vi "XY Graph Save Selected Plots Event.vi"(6 "Delimiter (TAB)":string="\t", 7 "X Axis Option (Dialog)":T1(ring), 8 "Error In":errorcluster, 9 "Save All Plots? (T)":bool=TRUE, 10 "File Path in":path, 11 "XYGraph Ref":T2) -> (0 "Error Out":errorcluster, 1 "Message":string, 2 "File Path out":path, 3 "Saved Plot Names":string[](array[string]), 4 "Saved Plot Indices":i32[](array[numeric]), 5 "Graph Name":string)   [LabVIEW 2021, in "XY Graph Add-Ons.lvlib"]
uses:
  XY Graph Add-Ons.lvlib
  XY Graph Refnum.ctl
  <userlib>/_OpenG.lib/array/array.llb/Index 1D Array Elements (Variant)__ogtk.vi
  <userlib>/_OpenG.lib/string/string.llb/openg_string.lvlib
  Strings/Strings.lvlib
  <userlib>/_OpenG.lib/array/array.llb/openg_array.lvlib
  GUI/GUI.lvlib
  Files/Files.lvlib
  Utilities/Utilities.lvlib
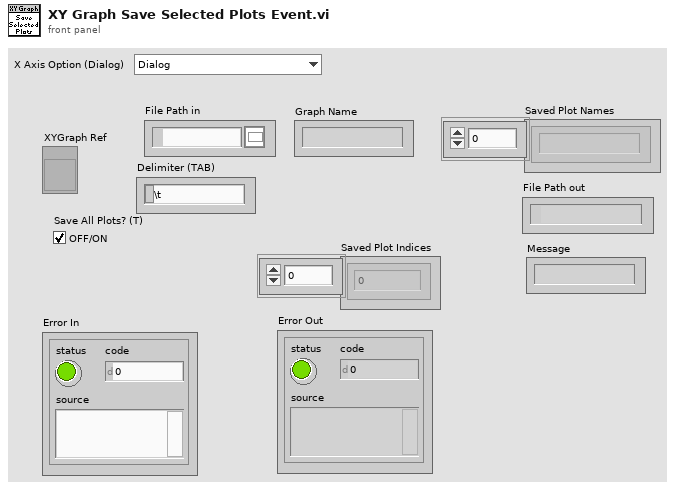
[diagram p1: front panel]
types:
  T1 = enum16{"Dialog", "Save Single X Axis if Common", "Save X Axis for each Plot"}
  T2 = typedef "XY Graph Add-Ons.lvlib/XY Graph Refnum.ctl" = refnum<vi>
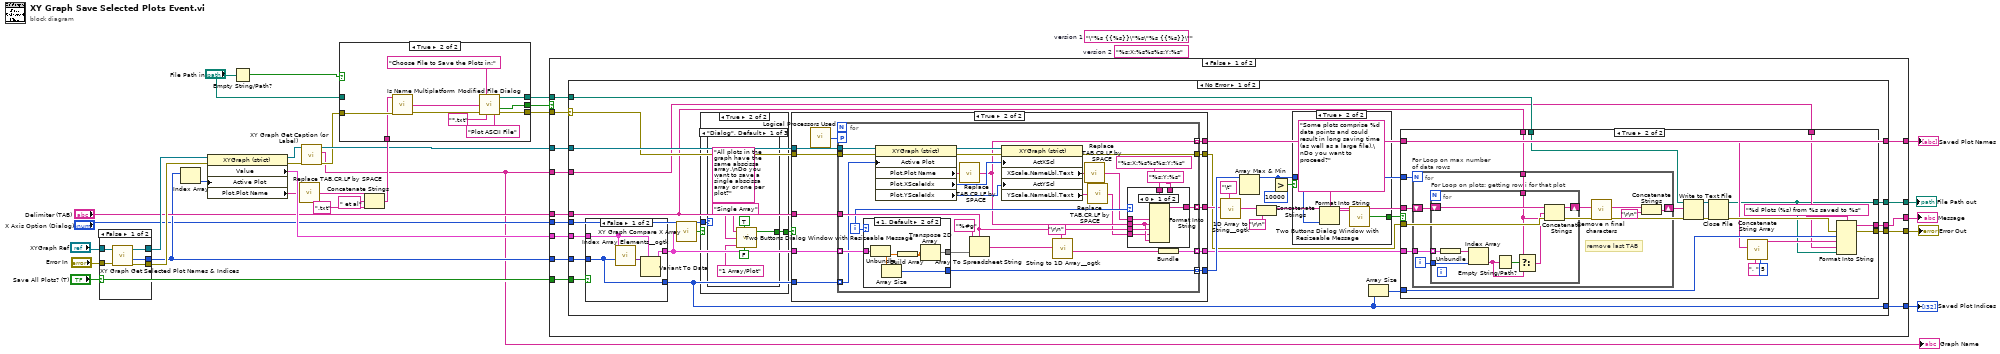
[diagram p0: block diagram]
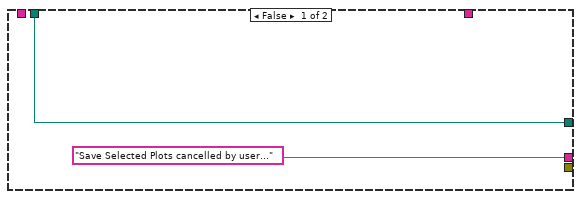
[diagram p2: hidden frame]
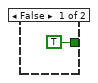
[diagram p3: hidden frame]
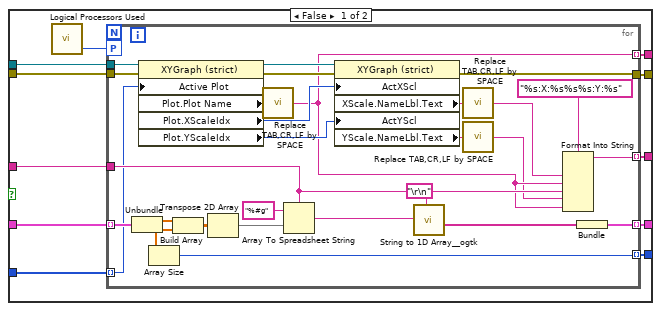
[diagram p4: hidden frame]
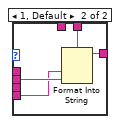
[diagram p5: hidden frame]
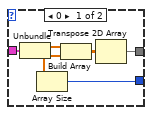
[diagram p6: hidden frame]
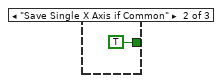
[diagram p8: hidden frame]
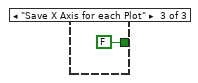
[diagram p9: hidden frame]
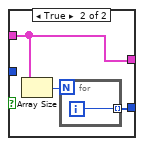
[diagram p10: hidden frame]
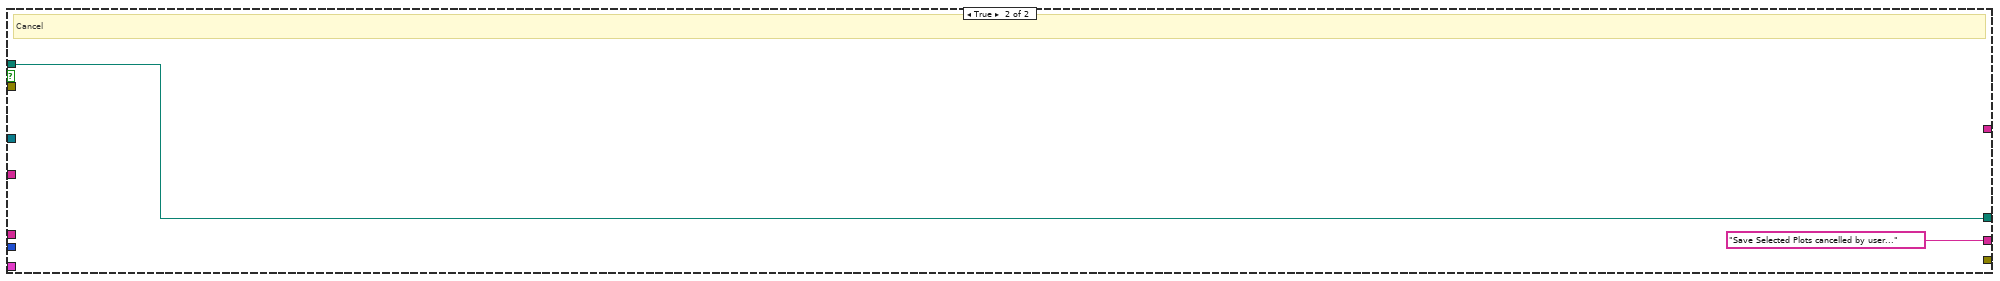
[diagram p12: hidden frame]
diagram:
  (unwired) "%s:X:%s%s%s:Y:%s"  # version 2
  (unwired) "\"%s {{%s}}\"%s\"%s {{%s}}\""  # version 1
  n1 = case shown="False" "Save All Plots? (T)" {
    tunnel: "XYGraph Ref" -> [w35 w37]
    tunnel: "Error In" -> [w34 w36]
    tunnel: [w33 w37] -> w28
    tunnel: [w32 _] -> w16
    tunnel: [w31 w36] -> w23
    frame False {
      n2 = call "XY Graph Get Selected Plot Names & Indices.vi"("error in (no error)"=w34, "XYGraph in"=w35) -> ("error out"=w31:errorcluster, "Selected Plots"=w32:i32[], "XYGraph out"=w33:T2)  [unwired: 5 in, 2 out]
    }
    frame True {
    }
  }
  n3 = Index Array(array=w16) -> (element=w15:i32)  [unwired: 1 in]
  n4 = property class="XYGraph (strict)"(reference=w28, error in=w23, "Active Plot"=w15) -> (reference out=w26:T2, error out=w5:errorcluster, "Value"=w27:cluster{"X Array":dbl[], "Y Array":dbl[]}[], "Plot.Plot Name"=w14:string)
  n5 = Empty String/Path?(string/path="File Path in") -> (empty?=w10:bool)
  n6 = call "Replace TAB,CR,LF by SPACE.vi"("String"=w14) -> ("String with replacements"=w1:string)  [unwired: 8 in]
  n7 = call "XY Graph Get Caption (or Label).vi"("error in (no error)"=w5, "XYGraph in"=w26) -> ("error out"=w4:errorcluster, "Caption (or Label) Text"=w3:string, "XYGraph out"=w6:T2)  [unwired: 7 in]
  "Graph Name" <- w3
  n8 = Concatenate Strings(w1, " et al" ("string"), ".txt" ("string")) -> (w11:string)
  n9 = case shown="True" w10 {
    tunnel: [w38 w49] -> w22
    tunnel: [w39 w48] -> w21
    tunnel: w4 -> [w38 w47]
    tunnel: w11 -> [_ w45]
    tunnel: "File Path in" -> [w39 _]
    tunnel: [_ w43] -> w2
    frame False {
    }
    frame True {
      n10 = call <vilib>:"Is Name Multiplatform.vi"("error in (no error)"=w47, "filename"=w45) -> ("error out"=w46:errorcluster, "suggested filename"=w44:string)  [unwired: 5 in, 3 out]
      n11 = call "Modified File Dialog.vi"("prompt"="Choose File to Save the Plots in:", "suggested filename"=w44, "error in (no error)"=w46, "pattern"="*.txt" ("pattern (all files)"), "pattern label"="Plot ASCII File") -> ("selected path"=w48:path, "Cancelled"=w43:bool, "error out"=w49:errorcluster)  [unwired: 7 in, 1 out]
    }
  }
  n12 = case shown="False" w2 {
    tunnel: w27 -> [w63 _]
    tunnel: [w62 _] -> w25
    tunnel: [w61 _] -> w24
    tunnel: w22 -> [w60 _]
    tunnel: w21 -> [w59 w257]
    tunnel: [w58 w257] -> w20
    tunnel: "Save All Plots? (T)" -> [w57 _]
    tunnel: [w56 _] -> w18
    tunnel: "Delimiter (TAB)" -> [w55 _]
    tunnel: w16 -> [w54 _]
    tunnel: "X Axis Option (Dialog)" -> [w53 _]
    tunnel: [w52 "Save Selected Plots cancelled by user..."] -> w7
    tunnel: w6 -> [w51 _]
    tunnel: w3 -> [w50 _]
    frame False {
      n13 = case shown="No Error" w60 {
        selector: w60 -> [w89 w255]
        tunnel: w63 -> [w93 _]
        tunnel: w51 -> [w92 _]
        tunnel: [w65 _] -> w62
        tunnel: [w70 w255] -> w61
        tunnel: w54 -> [w82 _]
        tunnel: w59 -> [w71 _]
        tunnel: [w69 _] -> w58
        tunnel: w57 -> [w83 _]
        tunnel: [w68 _] -> w56
        tunnel: w55 -> [w81 _]
        tunnel: w53 -> [w77 _]
        tunnel: [w66 _] -> w52
        tunnel: w50 -> [w64 _]
        frame No Error {
          n14 = case shown="False" w83 {
            tunnel: w93 -> [w249 w253]
            tunnel: [w248 w253] -> w80
            tunnel: w82 -> [w247 _]
            tunnel: [w247 w251] -> w68
            frame False {
              n15 = call-poly <userlib>:"Index Array Elements__ogtk.vi"("indices"=w247, "array"=w249) -> ("elements"=w250:variant[])  [unwired: 9 in]
              n16 = Variant To Data(type=w249, Variant=w250) -> (data=w248:cluster{"X Array":dbl[], "Y Array":dbl[]}[])  [unwired: 1 in, 1 out]
            }
            frame True {
              n17 = Array Size(array=w253) -> (size(s)=w252:i32)
              n18 = for {
                N: w252 -> [_]
                tunnel: [w254] -> w251 mode=indexing
                i -> [w254]
              }
            }
          }
          n19 = call "XY Graph Compare X Array.vi"("Plot Array"=w80) -> ("Same [X]?"=w79:bool)  [unwired: 8 in]
          n20 = case shown="True" w79 {
            selector: w79 -> [w236 _]
            tunnel: [w236 w238] -> w78
            tunnel: w77 -> [_ w237]
            frame False {
            }
            frame True {
              n21 = case shown="\"Dialog\", Default" w237 {
                tunnel: [w241 TRUE ("T button?") FALSE ("T button?")] -> w238
                frame "Dialog", Default {
                  n22 = call "Two Buttons Dialog Window with Resizeable Message.vi"("Message"="All plots in the graph have the same abscissa array.\nDo you want to save a single abscissa array or one per plot?" ("message"), "Return =  OK (T)"=TRUE, "OK Button Text"="Single Array" ("T button name (\"OK\")"), "Cancel Button Text"="1 Array/Plot" ("F button name (\"Cancel\")"), "ESC =  Cancel (T)"=FALSE) -> ("OK?"=w241:bool)  [unwired: 4 in]
                }
                frame "Save Single X Axis if Common" {
                }
                frame "Save X Axis for each Plot" {
                }
              }
            }
          }
          n23 = case shown="True" w78 {
            tunnel: w92 -> [w148 w187]
            tunnel: [w147 w186] -> w65
            tunnel: [w146 w185] -> w91
            tunnel: [w145 w184] -> w90
            tunnel: w89 -> [w144 w183]
            tunnel: [w143 w182] -> w88
            tunnel: [w142 w181] -> w72
            tunnel: w81 -> [w141 w180]
            tunnel: w68 -> [w140 w179]
            tunnel: w80 -> [w139 w178]
            frame False {
              n24 = call "Logical Processors Used.vi"() -> ("# Logical Processor Used"=w138:i32)  [unwired: 6 in]
              n25 = for {
                tunnel: w139 -> [w176] mode=indexing
                tunnel: w148 -> [w175]
                tunnel: [w151] -> w147 mode=indexing
                tunnel: w144 -> [w174]
                tunnel: [w167] -> w142
                tunnel: [w157] -> w145 mode=indexing
                tunnel: [w161] -> w146 mode=indexing
                tunnel: [w163] -> w143 mode=indexing
                workers-P: w138 -> [_]
                tunnel: w141 -> [w156]
                tunnel: w140 -> [w152] mode=indexing
                n26 = Unbundle(w176) -> ("X Array"=w169:dbl[], "Y Array"=w162:dbl[])
                n27 = property class="XYGraph (strict)"(reference=w175, error in=w174, "Active Plot"=w152) -> (reference out=w173:T2, error out=w168:errorcluster, "Plot.Plot Name"=w155:string, "Plot.XScaleIdx"=w166:u32, "Plot.YScaleIdx"=w165:u32)
                n28 = Array Size(array=w162) -> (size(s)=w161:i32)
                n29 = Build Array(w169, w162) -> (w172:dbl[][])
                n30 = Transpose 2D Array(2D array=w172) -> (transposed array=w171:dbl[][])
                n31 = call "Replace TAB,CR,LF by SPACE.vi"("String"=w155) -> ("String with replacements"=w151:string)  [unwired: 8 in]
                n32 = Array To Spreadsheet String(delimiter (Tab)=w156, array=w171, 3:"%#g" ("format string")) -> (spreadsheet string=w159:string)
                n33 = property class="XYGraph (strict)"(reference=w173, error in=w168, "ActXScl"=w166, "ActYScl"=w165) -> (error out=w167:errorcluster, "XScale.NameLbl.Text"=w154:string, "YScale.NameLbl.Text"=w153:string)  [unwired: 1 out]
                n34 = call <userlib>:"String to 1D Array__ogtk.vi"("delimiter (Tab)"="\r\n", "string"=w159) -> ("Array of Strings"=w158:string[])  [unwired: 9 in]
                n35 = call "Replace TAB,CR,LF by SPACE.vi"("String"=w154) -> ("String with replacements"=w150:string)  [unwired: 8 in]
                n36 = call "Replace TAB,CR,LF by SPACE.vi"("String"=w153) -> ("String with replacements"=w149:string)  [unwired: 8 in]
                n37 = Format Into String(format string="%s:X:%s%s%s:Y:%s", w150, w151, w156, w149, w151) -> (resulting string=w163:string)  [unwired: 2 in, 1 out]
                n38 = Bundle("Array of Strings"=w158) -> (w157:cluster{"Array of Strings":string[]})  [unwired: 1 in]
              }
            }
            frame True {
              n39 = call "Logical Processors Used.vi"() -> ("# Logical Processor Used"=w177:i32)  [unwired: 6 in]
              n40 = for {
                tunnel: w178 -> [w214] mode=indexing
                tunnel: w187 -> [w213]
                tunnel: [w190] -> w186 mode=indexing
                tunnel: w183 -> [w212]
                tunnel: [w207] -> w181
                tunnel: [w198] -> w184 mode=indexing
                tunnel: [w202] -> w185 mode=indexing
                tunnel: [w203] -> w182 mode=indexing
                workers-P: w177 -> [_]
                tunnel: w180 -> [w197]
                tunnel: w179 -> [w193] mode=indexing
                i -> [w192]
                n41 = case shown="1, Default" w192 {
                  tunnel: w214 -> [w230 w235]
                  tunnel: [w228 w233] -> w210
                  tunnel: [w225 w231] -> w202
                  frame 0 {
                    n42 = Unbundle(w230) -> ("X Array"=w227:dbl[], "Y Array"=w226:dbl[])
                    n43 = Array Size(array=w226) -> (size(s)=w225:i32)
                    n44 = Build Array(w227, w226) -> (w229:dbl[][])
                    n45 = Transpose 2D Array(2D array=w229) -> (transposed array=w228:dbl[][])
                  }
                  frame 1, Default {
                    n46 = Unbundle(w235) -> ("Y Array"=w232:dbl[])  [unwired: 1 out]
                    n47 = Array Size(array=w232) -> (size(s)=w231:i32)
                    n48 = Build Array(w232) -> (w234:dbl[][])
                    n49 = Transpose 2D Array(2D array=w234) -> (transposed array=w233:dbl[][])
                  }
                }
                n50 = property class="XYGraph (strict)"(reference=w213, error in=w212, "Active Plot"=w193) -> (reference out=w211:T2, error out=w208:errorcluster, "Plot.Plot Name"=w196:string, "Plot.XScaleIdx"=w206:u32, "Plot.YScaleIdx"=w205:u32)
                n51 = call "Replace TAB,CR,LF by SPACE.vi"("String"=w196) -> ("String with replacements"=w190:string)  [unwired: 8 in]
                n52 = Array To Spreadsheet String(delimiter (Tab)=w197, array=w210, 3:"%#g" ("format string")) -> (spreadsheet string=w200:string)
                n53 = property class="XYGraph (strict)"(reference=w211, error in=w208, "ActXScl"=w206, "ActYScl"=w205) -> (error out=w207:errorcluster, "XScale.NameLbl.Text"=w195:string, "YScale.NameLbl.Text"=w194:string)  [unwired: 1 out]
                n54 = call <userlib>:"String to 1D Array__ogtk.vi"("delimiter (Tab)"="\r\n", "string"=w200) -> ("Array of Strings"=w199:string[])  [unwired: 9 in]
                n55 = call "Replace TAB,CR,LF by SPACE.vi"("String"=w195) -> ("String with replacements"=w189:string)  [unwired: 8 in]
                n56 = call "Replace TAB,CR,LF by SPACE.vi"("String"=w194) -> ("String with replacements"=w188:string)  [unwired: 8 in]
                n57 = case shown="0" w192 {
                  tunnel: "%s:X:%s%s%s:Y:%s" ("format string") -> [w220 _]
                  tunnel: [w219 w224] -> w203
                  tunnel: w197 -> [w218 _]
                  tunnel: w190 -> [w217 w223]
                  tunnel: w189 -> [w216 _]
                  tunnel: w188 -> [w215 w222]
                  tunnel: "%s:Y:%s" ("format string") -> [_ w221]
                  frame 0 {
                    n58 = Format Into String(format string=w220, w216, w217, w218, w215, w217) -> (resulting string=w219:string)  [unwired: 2 in, 1 out]
                  }
                  frame 1, Default {
                    n59 = Format Into String(format string=w221, w222, w223) -> (resulting string=w224:string)  [unwired: 2 in, 1 out]
                  }
                }
                n60 = Bundle("Array of Strings"=w199) -> (w198:cluster{"Array of Strings":string[]})  [unwired: 1 in]
              }
            }
          }
          n61 = call <userlib>:"1D Array to String__ogtk.vi"("delimiter (Tab)"="\t", "Array of Strings"=w88) -> ("delimited string"=w86:string)  [unwired: 9 in]
          n62 = Array Max & Min(array=w91) -> (max value=w74:i32)  [unwired: 3 out]
          n63 = Concatenate Strings(w86, "\r\n") -> (w85:string)
          n64 = Greater?(x=w74, y=10000) -> (0:w75:bool)
          n65 = case shown="True" w75 {
            tunnel: [TRUE ("T button?") w135] -> w73
            tunnel: w74 -> [_ w134]
            frame False {
            }
            frame True {
              n66 = Format Into String(format string="Some plots comprise %d data points and could result in long saving time (as well as a large file).\nDo you want to proceed?", w134) -> (resulting string=w136:string)  [unwired: 2 in, 1 out]
              n67 = call "Two Buttons Dialog Window with Resizeable Message.vi"("Message"=w136) -> ("OK?"=w135:bool)  [unwired: 8 in]
            }
          }
          n68 = Array Size(array=w68) -> (size(s)=w67:i32)
          n69 = case shown="True" w73 {
            tunnel: w90 -> [_ w115]
            tunnel: w85 -> [_ w114]
            tunnel: w81 -> [_ w113]
            tunnel: w74 -> [_ w112]
            tunnel: w72 -> [_ w111]
            tunnel: w71 -> [w95 w109]
            tunnel: [_ w102] -> w70
            tunnel: [w95 w96] -> w69
            tunnel: w67 -> [_ w101]
            tunnel: ["Save Selected Plots cancelled by user..." ("source") w99] -> w66
            tunnel: w65 -> [_ w98]
            tunnel: w64 -> [_ w97]
            frame False {
            }
            frame True {
              n70 = for "For Loop on max number of data rows" {
                N: w112 -> [_]
                tunnel: w115 -> [w123]
                shift-right: [w119] -> w110
                shift-left: w114 -> [w122]
                tunnel: w113 -> [w116]
                i -> [w121]
                # "remove last TAB"
                n71 = for "For Loop on plots: getting row i for that plot" {
                  tunnel: w123 -> [w132] mode=indexing
                  shift-right: [w125] -> w120
                  shift-left: w122 -> [w127]
                  tunnel: w121 -> [w130]
                  tunnel: w116 -> [w124]
                  n72 = Unbundle(w132) -> ("Array of Strings"=w131:string[])
                  n73 = Index Array(array=w131, index=w130) -> (element=w128:string)
                  n74 = Empty String/Path?(string/path=w128) -> (empty?=w129:bool)
                  n75 = Select(t=w124, s=w129, f=w128) -> (s? t:f=w126:string)
                  n76 = Concatenate Strings(w127, w126, w124) -> (w125:string)
                }
                n77 = call "Remove n final characters.vi"("String in"=w120) -> ("String out"=w117:string)  [unwired: 8 in]
                n78 = Concatenate Strings(w117, "\r\n") -> (w119:string)
              }
              n79 = Write to Text File(file (use dialog)=w109, text=w110, error in=w111) -> (refnum out=w107:refnum<file>, error out=w108:errorcluster)  [unwired: 1 in, 1 out]
              n80 = Close File(refnum=w107, error in=w108) -> (path=w96:path, error out=w103:errorcluster)
              n81 = call "Concatenate String Array.vi"("Max Number of Elements (None: -1)"=5 ("Max Number of Elements (None: 1)"), "Separator (TAB)"=", ", "String Array"=w98) -> ("Formatted String"=w104:string)  [unwired: 8 in]
              n82 = Format Into String(format string="%d Plots (%s) from %s saved to %s", error in=w103, w101, w104, w97, w96) -> (resulting string=w99:string, error out=w102:errorcluster)  [unwired: 1 in]
            }
          }
        }
        frame Error {
        }
      }
    }
    frame True {
      # "Cancel"
    }
  }
  "Error Out" <- w24
  "Saved Plot Indices" <- w18
  "Saved Plot Names" <- w25
  "File Path out" <- w20
  "Message" <- w7
